vi "MKII.vi"() -> ()   [LabVIEW 2019]
panel:
  out "TESTER":bool
  out "FALLA PRESENTE":bool
  out "MAQUINA EN ORIGEN":bool
  out "RESET":bool
  in  "Tab Control":T1(tab)
  out "TESTER":bool
  in  "MOVER A ORIGEN":bool
  in  "MODO MANUAL":bool
  in  "MODO AUTOMATICO":bool
  out "EST 3":bool
  out "EST 2":bool
  out "EST 1":bool
  in  "HABILITAR ESTACION 3":bool
  in  "HABILITAR ESTACION 2":bool
  in  "HABILITAR ESTACION":bool
  out "VALOR OBTENIDO":dbl
  out "VALOR OBTENIDO":dbl
  out "VALOR OBTENIDO":dbl
  out "SOL SECADO":bool
  out "TORRETA ROJA":bool
  out "TORRETA AMBAR":bool
  out "TORRETA VERDE":bool
  out "BOMBA ENCENDIDA":bool
  out "SOL SECADO 1":bool
  out "SOL ARRIBA":bool
  out "SOL ABAJO":bool
  out "S. DETECTOR 2":bool
  out "SEÑAL CORTINA 2":bool
  out "SEÑAL CORTINA 1":bool
  out "BIMANUAL 2":bool
  out "BIMANUAL 1":bool
  out "S. DETECTOR 1":bool
  out "SOBRECARGA BOMBA":bool
  out "S. LIMITE ARRIBA":bool
  out "S. LIMITE ABAJO":bool
  in  "ESTADISTICAS DE PRODUCCION":bool
  in  "MANUAL":bool
  in  "CONFIGRUARCION DE PARAMETROS":bool
  in  "HISTORIAL DE FALLAS":bool
  in  "ENTRADAS Y SALIDAS":bool
  in  "PRODUCCIÓN":bool
  in  "MODO DE OPERACION 2":bool
  # "MENÚ PRINCIPAL"
  # "MODO DE OPERACIÓN"
  # "ESTACION 1"
  # "ESTACION 2"
  # "ESTACION 3"
  # "PRODUCCIÓN"
  # "ENTRADAS                        SALIDAS"
  # "CONFIGURACION DE PARAMETROS"
  # "MANUAL"
  # "ESTADISTICAS DE PRODUCCIÓN"
  # "HISTORIAL DE FALLAS"
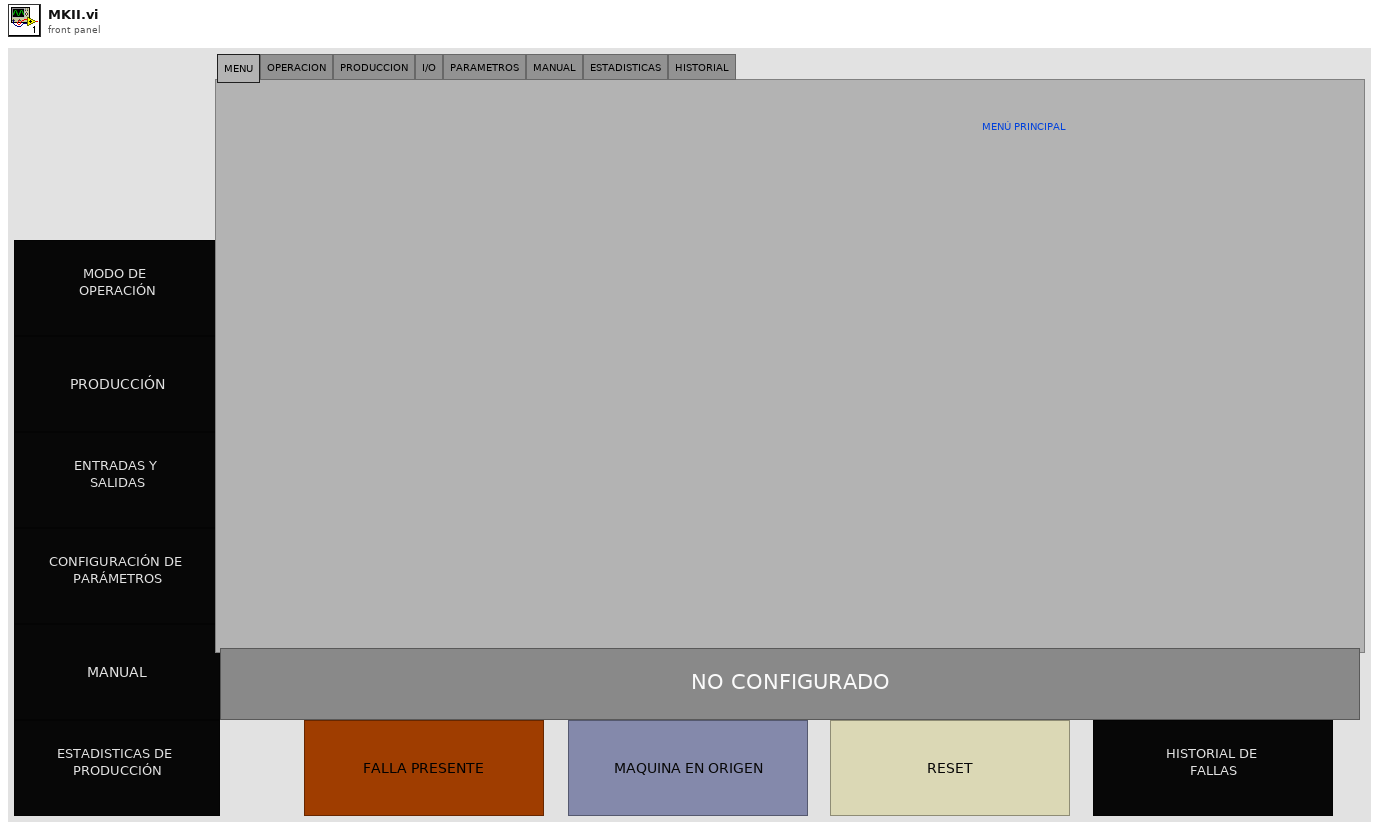
[diagram p1: front panel]
types:
  T1 = enum32{"MENU", "OPERACION", "PRODUCCION", "I/O", "PARAMETROS", "MANUAL", "ESTADISTICAS", "HISTORIAL"}
  T2 = enum32{"MENU", "OPERACION", "PRODUCCION", "I/O", "PARAMETROS", "MANUAL", "ESTADISTICAS", "FALLAS"}
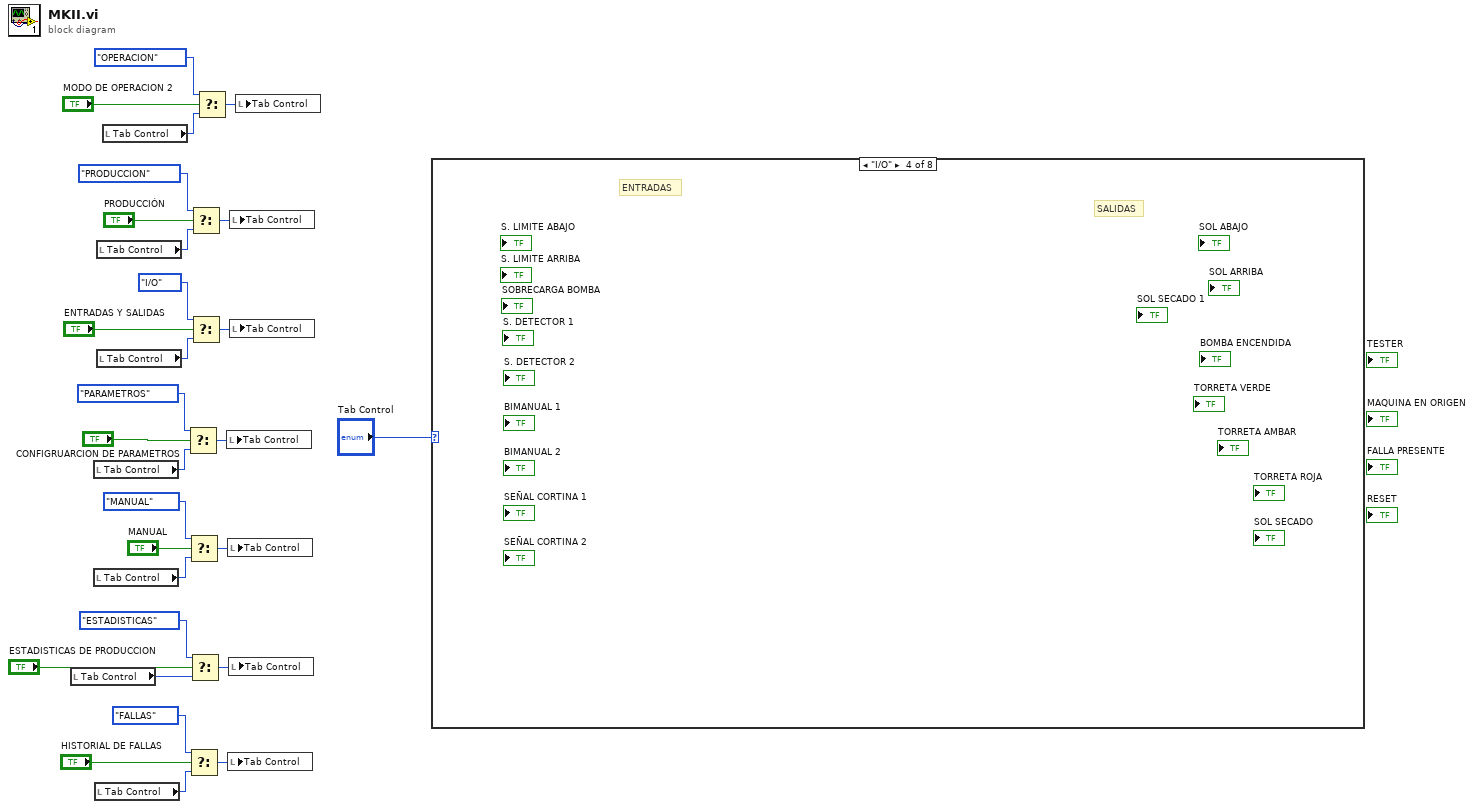
[diagram p0: block diagram]
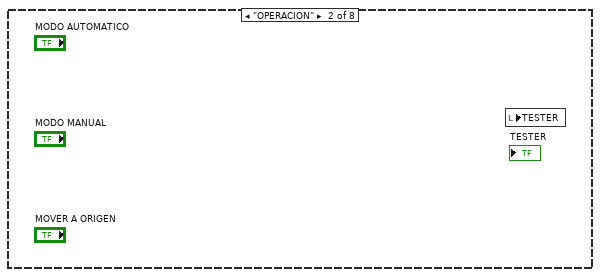
[diagram p3: hidden frame]
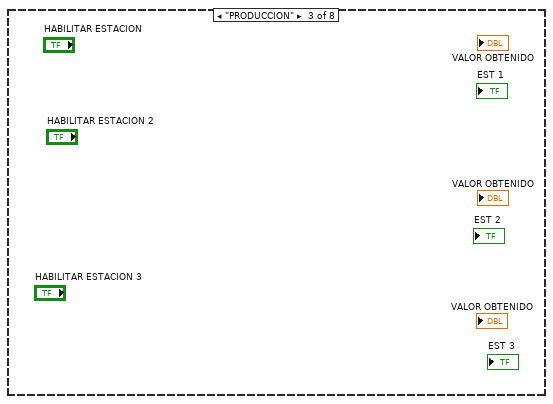
[diagram p4: hidden frame]
diagram:
  n1 = local read "Tab Control"() -> (w14:T1)
  n2 = local read "Tab Control"() -> (w21:T1)
  n3 = local read "Tab Control"() -> (w18:T1)
  n4 = local read "Tab Control"() -> (w17:T1)
  n5 = local read "Tab Control"() -> (w23:T1)
  n6 = local read "Tab Control"() -> (w22:T1)
  n7 = local read "Tab Control"() -> (w27:T1)
  n8 = Select(t=T2."PARAMETROS" ("Tab Control"), s="CONFIGRUARCION DE PARAMETROS", f=w21) -> (s? t:f=w20:u32)
  n9 = Select(t=T2."MANUAL" ("Tab Control"), s="MANUAL", f=w18) -> (s? t:f=w19:u32)
  n10 = Select(t=T2."FALLAS" ("Tab Control"), s="HISTORIAL DE FALLAS", f=w17) -> (s? t:f=w16:u32)
  n11 = Select(t=T2."ESTADISTICAS" ("Tab Control"), s="ESTADISTICAS DE PRODUCCION", f=w14) -> (s? t:f=w15:u32)
  n12 = Select(t=T2."PRODUCCION" ("Tab Control"), s="PRODUCCIÓN", f=w23) -> (s? t:f=w25:u32)
  n13 = Select(t=T2."I/O" ("Tab Control"), s="ENTRADAS Y SALIDAS", f=w22) -> (s? t:f=w24:u32)
  n14 = Select(t=T2."OPERACION" ("Tab Control"), s="MODO DE OPERACION 2", f=w27) -> (s? t:f=w26:u32)
  n15 = local write "Tab Control"(w20) -> ()
  n16 = local write "Tab Control"(w19) -> ()
  n17 = local write "Tab Control"(w16) -> ()
  n18 = local write "Tab Control"(w15) -> ()
  n19 = local write "Tab Control"(w25) -> ()
  n20 = local write "Tab Control"(w24) -> ()
  n21 = local write "Tab Control"(w26) -> ()
  n22 = case shown="\"I/O\"" "Tab Control" {
    frame "MENU", Default {
    }
    frame "OPERACION" {
      n23 = local read "TESTER"() -> ()  [unwired: 1 in]
    }
    frame "PRODUCCION" {
    }
    frame "I/O" {
      # "SALIDAS"
      # "ENTRADAS"
    }
    frame "PARAMETROS" {
    }
    frame "MANUAL" {
    }
    frame "ESTADISTICAS" {
    }
    frame "HISTORIAL" {
    }
  }
